vi "TEST - CLIMBER.vi"(8 "error in (no error)":errorcluster, 10 "Cluster of JOYSTICK and CLIMBER ref info":T8, 11 "refnum name":string) -> (0 "error out":errorcluster)   [LabVIEW 2020]
uses:
  <vilib>/Rock Robotics/WPI/ThirdParty/Phoenix-LabVIEW/Motor Controller/Controls/CTRE_Phoenix_MotorControl_ControlMode.ctl
  <vilib>/Rock Robotics/WPI/Joystick/WPI_JoystickDeviceEnum.ctl
  <vilib>/Rock Robotics/WPI/Joystick/WPI_JoystickDevRef.ctl
  <vilib>/Rock Robotics/SystemInterfaces/DIO/FPGA_DIOPWMChannel.ctl
  <vilib>/Rock Robotics/WPI/PWM/WPI_PWMDeadband.ctl
  <vilib>/Rock Robotics/WPI/MotorControl/WPI_MotorControlType.ctl
  <vilib>/Rock Robotics/SystemInterfaces/DIO/FPGA_DIOChannel.ctl
  <vilib>/Rock Robotics/WPI/MotorControl/WPI_MotorControlDeviceRef.ctl
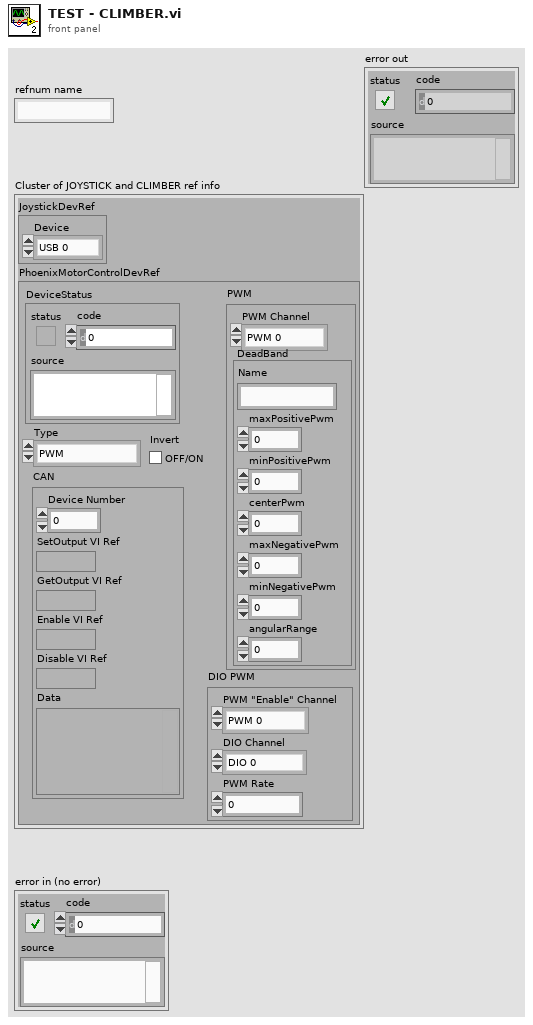
[diagram p1: front panel]
types:
  T1 = typedef "WPI_JoystickDevRef.ctl" = cluster{"Device":T2}
  T2 = typedef "WPI_JoystickDeviceEnum.ctl" = enum16{"USB 0", "USB 1", "USB 2", "USB 3", "USB 4", "USB 5"}
  T3 = typedef "WPI_MotorControlDeviceRef.ctl" = cluster{"DeviceStatus":errorcluster, "Type":T4, "PWM":cluster{"PWM Channel":T5, "DeadBand":T6}, "CAN":cluster{"Device Number":u8, "SetOutput VI Ref":variant, "GetOutput VI Ref":variant, "Enable VI Ref":variant, "Disable VI Ref":variant, "Data":variant}, "Invert":bool, "DIO PWM":cluster{"PWM \"Enable\" Channel":T5, "DIOChannel":T7, "PWM Rate":dbl}}
  T4 = typedef "WPI_MotorControlType.ctl" = enum16{"PWM", "CAN", "DIO PWM"}
  T5 = typedef "FPGA_DIOPWMChannel.ctl" = enum8{"PWM 0", "PWM 1", "PWM 2", "PWM 3", "PWM 4", "PWM 5", "PWM 6", "PWM 7", "PWM 8", "PWM 9", "PWM MXP 0", "PWM MXP 1", "PWM MXP 2", "PWM MXP 3", "PWM MXP 4", "PWM MXP 5", "PWM MXP 6", "PWM MXP 7", "PWM MXP 8", "PWM MXP 9", "Invalid"}
  T6 = typedef "WPI_PWMDeadband.ctl" = cluster{"Name":string, "maxPositivePwm":i32, "minPositivePwm":i32, "centerPwm":i32, "maxNegativePwm":i32, "minNegativePwm":i32, "angularRange":u16}
  T7 = typedef "FPGA_DIOChannel.ctl" = enum8{"DIO 0", "DIO 1", "DIO 2", "DIO 3", "DIO 4", "DIO 5", "DIO 6", "DIO 7", "DIO 8", "DIO 9", "DIO MXP 0", "DIO MXP 1", "DIO MXP 2", "DIO MXP 3", "DIO MXP 4", "DIO MXP 5", "DIO MXP 6", "DIO MXP 7", "DIO MXP 8", "DIO MXP 9", "DIO MXP 10", "DIO MXP 11", "DIO MXP 12", "DIO MXP 13", "DIO MXP 14", "DIO MXP 15", "SPI Port CS1", "SPI Port CS2", "SPI Port CS3", "SPI Port MISO", "SPI Port MOSI", "Invalid"}
  T8 = cluster{"JoystickDevRef":T1, "PhoenixMotorControlDevRef":T3}
  T9 = typedef "CTRE_Phoenix_MotorControl_ControlMode.ctl" = u16
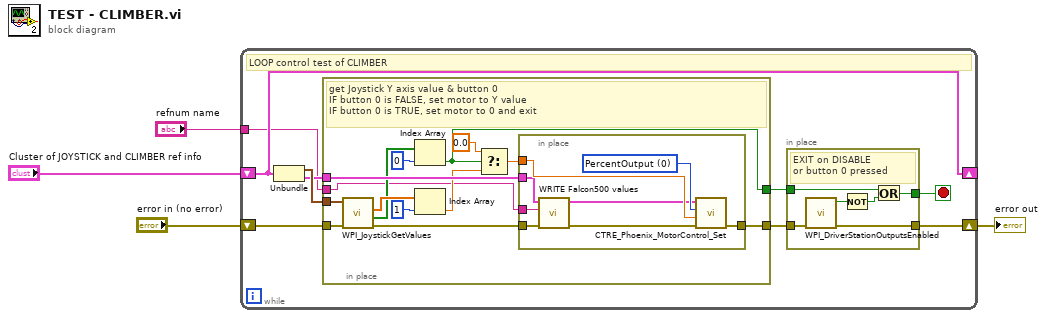
[diagram p0: block diagram]
diagram:
  n1 = while {
    shift-right: [w13] -> _
    shift-left: "Cluster of JOYSTICK and CLIMBER ref info" -> [w13]
    tunnel: "refnum name" -> [w7]
    shift-right: [w6] -> w1
    shift-left: "error in (no error)" -> [w5]
    stop <- w10 stop-if-true
    # "LOOP control test of CLIMBER"
    n2 = Unbundle(w13) -> ("JoystickDevRef"=w12:T1, "PhoenixMotorControlDevRef"=w11:T3)
    n3 = in-place {
      in-place-border: w12 -> [w27]
      in-place-border: w11 -> [w25]
      in-place-border: [w19] -> w9
      in-place-border: [w16] -> w8
      in-place-border: w5 -> [w15]
      in-place-border: w7 -> [w14]
      # "get Joystick Y axis value & button 0\nIF button 0 is FALSE, set motor to Y value\nIF button 0 is TRUE, set motor to 0 and exit"
      n4 = call <vilib>:"WPI_JoystickGetValues.vi"("error in (no error)"=w15, "JoystickDevRef"=w27) -> ("error out"=w26:errorcluster, "Buttons"=w22:bool[], "Axes"=w24:dbl[])  [unwired: 5 in, 2 out]
      n5 = Index Array(array=w22, index=0) -> (element=w19:bool)
      n6 = Index Array(array=w24, index=1) -> (element=w18:dbl)
      n7 = Select(t=0.0, s=w19, f=w18) -> (s? t:f=w20:dbl)
      n8 = in-place {
        in-place-border: w26 -> [w31]
        in-place-border: w25 -> [w30]
        in-place-border: w20 -> [w34]
        in-place-border: [w33] -> w16
        in-place-border: w14 -> [w28]
        w35 = T9 0 items=["PercentOutput"=0, "Position"=1, "Velocity"=2, "Current"=3, "Follower"=5, "MotionProfile"=6, "MotionMagic"=7, "MotionProfileArc"=10, "Disabled"=15] ("Control Mode")
        n9 = call "WRITE Falcon500 values.vi"("PhoenixMotorControlDevRef"=w30, "refnum name"=w28, "error in (no error)"=w31) -> ("PhoenixMotorControlDevRef 2"=w29:T3, "error out"=w32:errorcluster)  [unwired: 5 in]
        n10 = call <vilib>:"CTRE_Phoenix_MotorControl_Set.vi"("error in (no error)"=w32, "Output"=w34, "Control Mode"=w35, "PhoenixMotorControlDevRef"=w29) -> ("error out"=w33:errorcluster)  [unwired: 6 in, 1 out]
      }
    }
    n11 = in-place {
      in-place-border: [w39] -> w10
      in-place-border: w9 -> [w38]
      in-place-border: w8 -> [w37]
      in-place-border: [w36] -> w6
      # "EXIT on DISABLE\nor button 0 pressed"
      n12 = call <vilib>:"WPI_DriverStationOutputsEnabled.vi"("error in"=w37) -> ("error out"=w36:errorcluster, "OutputsEnabled?"=w41:bool)  [unwired: 9 in]
      n13 = Not(x=w41) -> (.not. x?=w40:bool)
      n14 = Or(x=w38, y=w40) -> (x .or. y?=w39:bool)
    }
  }
  "error out" <- w1
